vi "Get Version Info.vi"() -> (1 "Expt VIs Version out":i32, 2 "Version Info":string)   [LabVIEW 2020]
uses:
  <resource>/objmgr/daqmx.rc
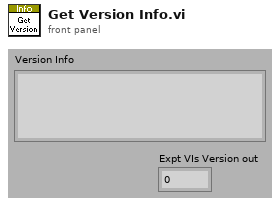
[diagram p1: front panel]
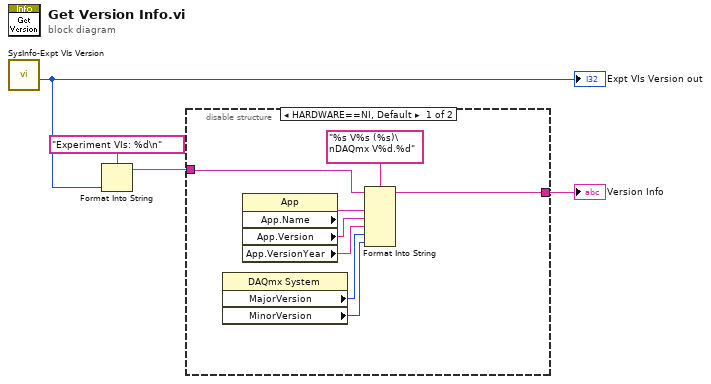
[diagram p0: block diagram]
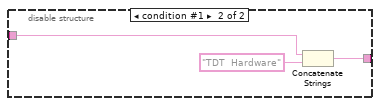
[diagram p2: hidden frame]
diagram:
  n1 = call "SysInfo-Expt VIs Version.vi"() -> ("Expt VIs Version out"=w1:i32)  [unwired: 11 in]
  "Expt VIs Version out" <- w1
  n2 = Format Into String(format string="Experiment VIs: %d\n", w1) -> (resulting string=w2:string)  [unwired: 2 in, 1 out]
  n3 = disable-structure shown="HARDWARE==NI, Default" {
    disable-tunnel: [w8 w15] -> w4
    disable-tunnel: w2 -> [w5 w14]
    frame condition #0 (active) {
      n4 = property class="DAQmx System"() -> ("MajorVersion"=w7:u32, "MinorVersion"=w6:u32)  [unwired: 2 in, 2 out]
      n5 = property class="App"() -> ("App.Name"=w11:string, "App.Version"=w10:string, "App.VersionYear"=w9:string)  [unwired: 2 in, 2 out]
      n6 = Format Into String(format string="%s V%s (%s)\nDAQmx V%d.%d", initial string=w5, w11, w10, w9, w7, w6) -> (resulting string=w8:string)  [unwired: 1 in, 1 out]
    }
    frame condition #1 {
      n7 = Concatenate Strings(w14, "TDT  Hardware" ("string")) -> (w15:string)
    }
  }
  "Version Info" <- w4
